vi "MSEncoder SubVI DynamicTimeout_Read.vi"(8 "error in (no error)":errorcluster, 11 "MSEncoder in":refnum<class "MSEncoder.lvclass">) -> (0 "error out":errorcluster, 2 "Timeout_ms":i32, 3 "MSEncoder out":refnum<class "MSEncoder.lvclass">)   [LabVIEW 2018, in "MSEncoder.lvclass"]
uses:
  MSEncoder.lvclass
  MSEncoder.lvclass/MSEncoder.ctl
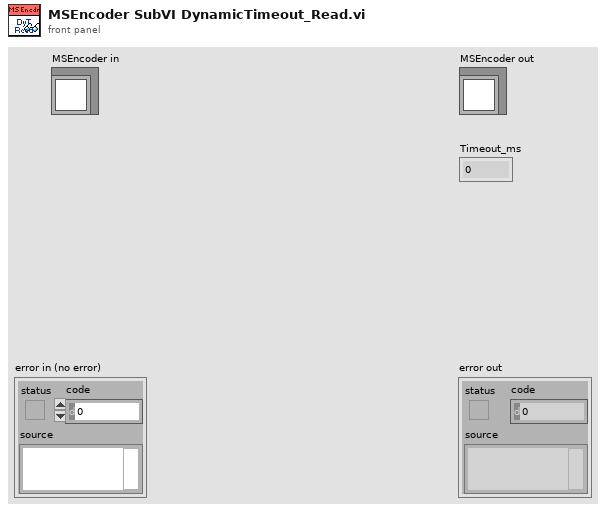
[diagram p1: front panel]
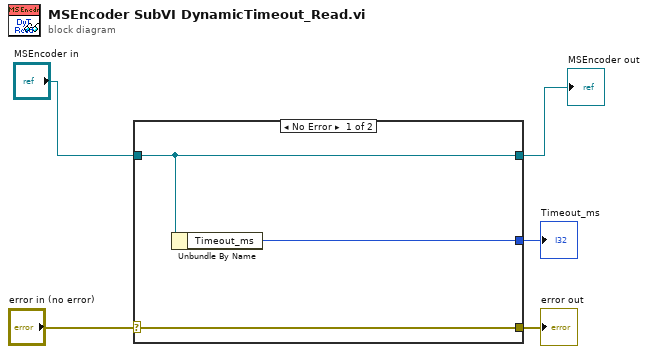
[diagram p0: block diagram]
diagram:
  n1 = case shown="No Error" "error in (no error)" {
    selector: "error in (no error)" -> [w8 w9]
    tunnel: [w8 w9] -> w4
    tunnel: [w7 w10] -> w1
    tunnel: "MSEncoder in" -> [w7 w10]
    tunnel: [w6 _] -> w3
    frame No Error {
      n2 = Unbundle By Name(w7) -> ("Timeout_ms"=w6:i32)
    }
    frame Error {
    }
  }
  "error out" <- w4
  "Timeout_ms" <- w3
  "MSEncoder out" <- w1
